vi "ModuloFractionArray.vi"(1 "Round Method (Nearest)":T1(ring)=enum."Round Nearest", 2 "Modulo Fraction":dbl=0.1 format="%#_13g", 3 "Input":dbl[](array[numeric]) format="%#_13g") -> (0 "Output":dbl[](array[numeric]) format="%#_13g")   [LabVIEW 2022 SP3]
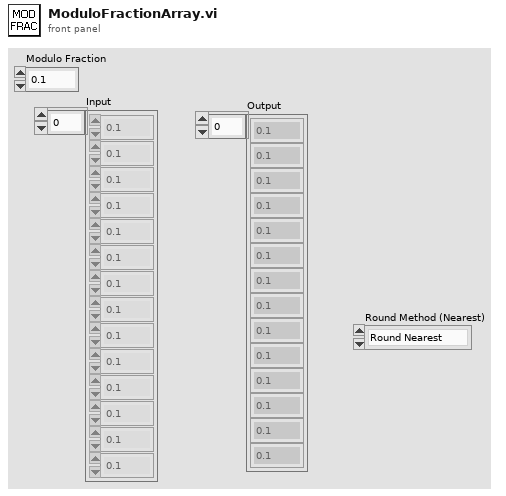
[diagram p1: front panel]
types:
  T1 = enum16{"Round to +INF", "Round Nearest", "Round to -INF"}
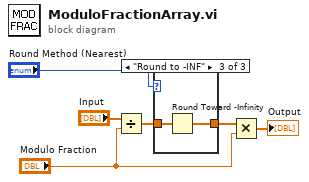
[diagram p0: block diagram]
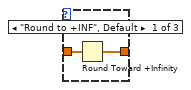
[diagram p2: hidden frame]
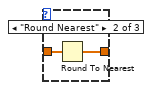
[diagram p3: hidden frame]
diagram:
  n1 = Divide(x="Input", y="Modulo Fraction") -> (x/y=w2:dbl[])
  n2 = case shown="\"Round to -INF\"" "Round Method (Nearest)" {
    tunnel: [w7 w9 w11] -> w1
    tunnel: w2 -> [w8 w10 w12]
    frame "Round to +INF", Default {
      n3 = Round Toward +Infinity(x=w8) -> (ceil(x): smallest int >= x=w7:dbl[])
    }
    frame "Round Nearest" {
      n4 = Round To Nearest(number=w10) -> (nearest integer value=w9:dbl[])
    }
    frame "Round to -INF" {
      n5 = Round Toward -Infinity(1:w12) -> (0:w11:dbl[])
    }
  }
  n6 = Multiply(x=w1, y="Modulo Fraction") -> (x*y=→"Output":dbl[])
